vi "Snap Image.vi"(8 "error in (no error)":errorcluster, 11 "Bobcat 640 in":refnum<class "Bobcat 640.lvclass">) -> (0 "error out":errorcluster, 3 "Bobcat 640 out":refnum<class "Bobcat 640.lvclass">)   [LabVIEW 2018, in "Bobcat 640.lvlib" / "Bobcat 640.lvclass"]
uses:
  Bobcat 640.lvclass
  Bobcat 640.lvclass/Bobcat 640.ctl
  PPLs/Camera/Parent/Camera.lvlibp/Camera.lvclass
  <vilib>/vision/driver/NI_Vision_Acquisition_Software.lvlib
  C:/AME Test Engineering/LabVIEW/PPLs/Camera/Parent/Camera.lvlibp/Camera.lvclass
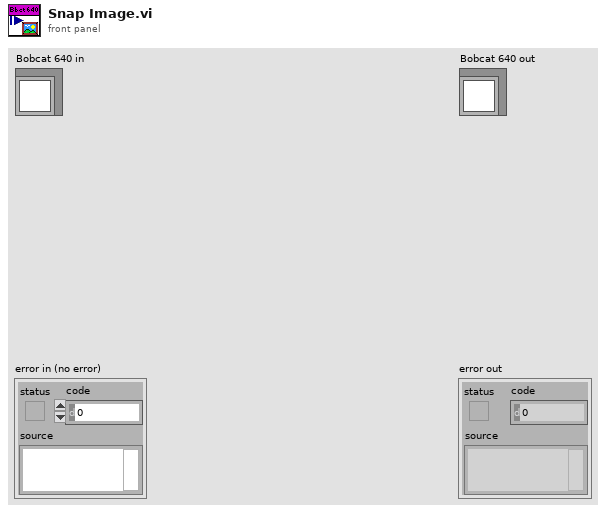
[diagram p1: front panel]
types:
  T1 = typedef "IMAQdx.ctl" = refnum<k21>
  T2 = typedef "Camera.lvlibp/IMAQ Image.ctl" = refnum<image>
  T3 = typedef "IMAQ Image.ctl" = refnum<image>
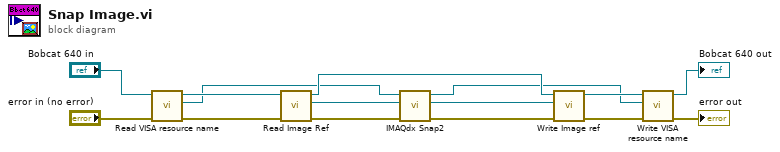
[diagram p0: block diagram]
diagram:
  n1 = call "Read VISA resource name.vi"("error in (no error)"="error in (no error)", "Bobcat 640 in"="Bobcat 640 in") -> ("error out"=w15:errorcluster, "IMAQdx Session"=w5:T1, "Bobcat 640 out"=w14:refnum<class "Bobcat 640.lvclass">)  [unwired: 7 in]
  n2 = call "Read Image Ref.vi"("error in (no error)"=w15, "Camera in"=w14) -> ("error out"=w4:errorcluster, "Image"=w6:T2, "Camera out"=w9:refnum<class "Bobcat 640.lvclass">)  [unwired: 7 in]
  n3 = call <vilib>:"IMAQdx Snap2.vi"("error in"=w4, "Image In"=w6, "Session In"=w5) -> ("error out"=w1:errorcluster, "Image Out"=w3:T3, "Session Out"=w2:T1)  [unwired: 6 in]
  n4 = call "Write Image ref.vi"("error in (no error)"=w1, "Image"=w3, "Camera in"=w9) -> ("error out"=w13:errorcluster, "Camera out"=w8:refnum<class "Bobcat 640.lvclass">)  [unwired: 7 in]
  n5 = call "Write VISA resource name.vi"("error in (no error)"=w13, "IMAQdx Session"=w2, "Bobcat 640 in"=w8) -> ("error out"=→"error out":errorcluster, "Bobcat 640 out"=→"Bobcat 640 out":refnum<class "Bobcat 640.lvclass">)  [unwired: 7 in]
